vi "信息流测试-使用控件（成功）.vi"() -> ()   [LabVIEW 2019, in "test.lvlib"]
uses:
  SubVI/test.lvlib
panel:
  in  "Resource In":refnum<visa-resource-name>
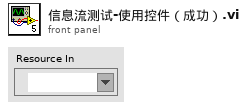
[diagram p1: front panel]
types:
  T1 = typedef "test.lvlib/控件 1.ctl" = cluster{i32, "数值 2":i32, "字符串":string, "布尔":bool, bool, "Resource In":refnum<visa-resource-name>, bool, string}
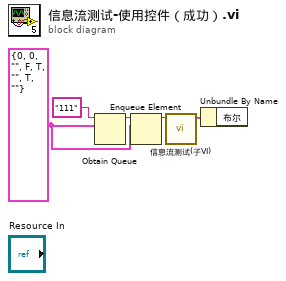
[diagram p0: block diagram]
diagram:
  w2 = T1 {0, "数值 2"=0, "字符串"="", "布尔"=FALSE, TRUE, "Resource In"="", TRUE, ""}
  n1 = Obtain Queue(name (unnamed)="111" ("名称（未命名）"), element data type=w2) -> (queue out=w5:refnum<queue>)  [unwired: 3 in, 2 out]
  n2 = Enqueue Element(queue=w5, element=w2) -> (queue out=w4:refnum<queue>)  [unwired: 2 in, 2 out]
  n3 = call "信息流测试(子VI).vi"("队列输入"=w4) -> ("簇"=w1:T1)  [unwired: 10 in]
  n4 = Unbundle By Name(w1) -> ()  [unwired: 1 out]
